vi "timestampAndDataToTable 4ch.vi"(7 "show time left [F]":bool, 9 "device type [AB1004]":T2=1004 items=["any"=0, "AB1002"=1002, "AB1004"=1004], 10 "data in":T4(array[cluster]), 11 "session start timestamp":timestamp) -> (1 "table data":string[][](array[string]), 2 "table headers":string[](array[string]), 3 "read timestamp":timestamp[](array[timestamp]))   [LabVIEW 2015]
doc: "Arranges data from queue in a 2D string array to be written or displayed as a table.\nData from queue is an array with counter4ch data clusters and their timestamps.\nRemoves the time_left column if requested."
uses:
  <instrlib>/Tausand AB1000/Public/Controls/counters4ch.ctl
  <instrlib>/Tausand AB1000/Public/Controls/deviceTypeRing.ctl
  <instrlib>/Tausand AB1000/Public/Controls/counters2ch.ctl
  <instrlib>/Tausand AB1000/Tausand AB1000.lvlib
panel:
  out "col index to remove":i32[](array[numeric])
  out "erase this col":bool
  in  "counters":T1
  out "time from begin in s":string[](array[string])
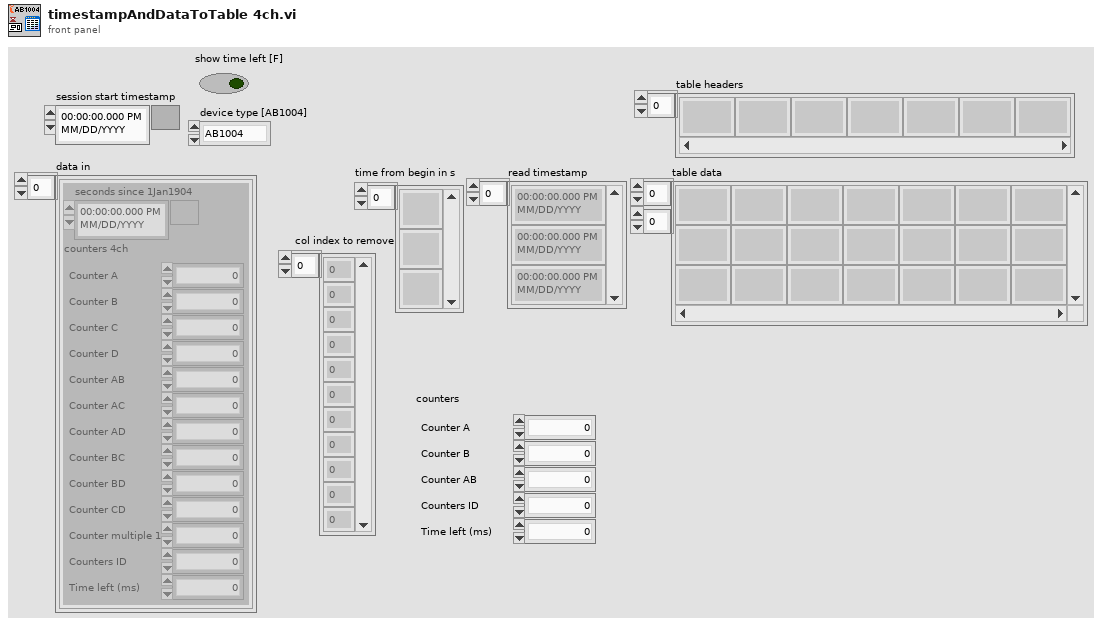
[diagram p1: front panel]
types:
  T1 = typedef "Tausand AB1000.lvlib/counters2ch.ctl" = cluster{"counter_A":u32, "counter_B":u32, "counter_AB":u32, "counters_ID":u32, "time_left":u32}
  T2 = typedef "Tausand AB1000.lvlib/deviceTypeRing.ctl" = u16
  T3 = typedef "Tausand AB1000.lvlib/counters4ch.ctl" = cluster{"counter_A":u32, "counter_B":u32, "counter_C":u32, "counter_D":u32, "counter_AB":u32, "counter_AC":u32, "counter_AD":u32, "counter_BC":u32, "counter_BD":u32, "counter_CD":u32, "counter_multiple_1":u32, "counters_ID":u32, "time_left":u32}
  T4 = cluster{"seconds since 1Jan1904":timestamp, "counters 4ch":T3}[]
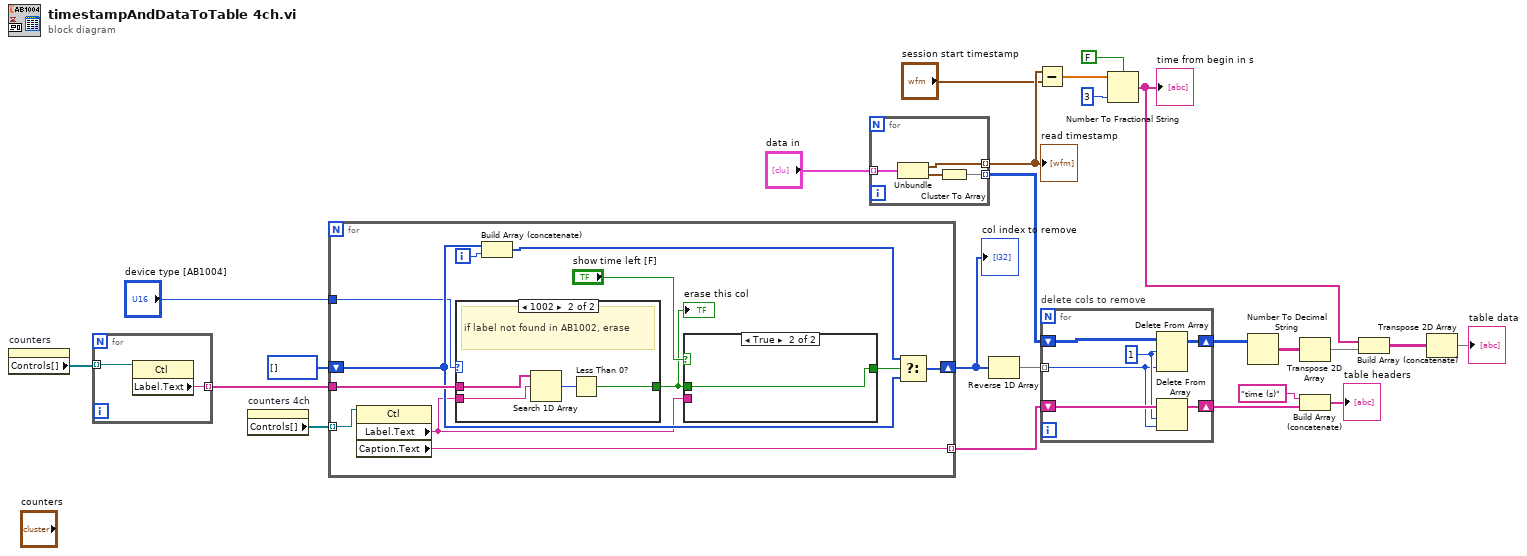
[diagram p0: block diagram]
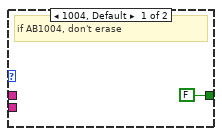
[diagram p2: hidden frame]
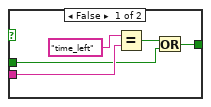
[diagram p3: hidden frame]
diagram:
  n1 = property on="counters" class="Clust (strict)"() -> ("Controls[]"=w1:refnum<vi>[])  [unwired: 2 in, 2 out]
  n2 = for {
    tunnel: w1 -> [w26] mode=indexing
    tunnel: [w25] -> w10 mode=indexing
    n3 = property class="Ctl"(reference=w26) -> ("Label.Text"=w25:string)  [unwired: 1 in, 2 out]
  }
  n4 = property on="counters 4ch" class="Clust (strict)"() -> ("Controls[]"=w15:refnum<vi>[])  [unwired: 2 in, 2 out]
  n5 = for {
    tunnel: w15 -> [w38] mode=indexing
    tunnel: [w27] -> w4 mode=indexing
    tunnel: w10 -> [w37]
    shift-right: [w33] -> w7
    shift-left: i32[] [] -> [w34]
    tunnel: "device type [AB1004]" -> [w29]
    i -> [w36]
    n6 = property class="Ctl"(reference=w38) -> ("Label.Text"=w28:string, "Caption.Text"=w27:string)  [unwired: 1 in, 2 out]
    n7 = case shown="1002" w29 {
      tunnel: w37 -> [_ w43]
      tunnel: w28 -> [_ w41]
      tunnel: [FALSE w40] -> w31
      frame 1004, Default {
        # "if AB1004, don't erase"
      }
      frame 1002 {
        # "if label not found in AB1002, erase"
        n8 = Search 1D Array(1D array=w43, element=w41) -> (index of element=w42:i32)  [unwired: 1 in]
        n9 = Less Than 0?(x=w42) -> (x < 0?=w40:bool)
      }
    }
    "erase this col" <- w31
    n10 = Build Array (concatenate)(w34, w36) -> (w35:i32[])
    n11 = case shown="True" "show time left [F]" {
      tunnel: w28 -> [w48 _]
      tunnel: [w44 w49] -> w30
      tunnel: w31 -> [w45 w49]
      frame False {
        n12 = Equal?(x="time_left" ("element"), y=w48) -> (x = y?=w46:bool)
        n13 = Or(x=w46, y=w45) -> (x .or. y?=w44:bool)
      }
      frame True {
      }
    }
    n14 = Select(t=w35, s=w30, f=w34) -> (s? t:f=w33:i32[])
  }
  "col index to remove" <- w7
  n15 = for {
    tunnel: "data in" -> [w53] mode=indexing
    tunnel: [w52] -> w22 mode=indexing
    tunnel: [w51] -> w8 mode=indexing
    n16 = Unbundle(w53) -> ("seconds since 1Jan1904"=w52:timestamp, "counters 4ch"=w50:T3)
    n17 = Cluster To Array(cluster=w50) -> (array=w51:u32[])
  }
  "read timestamp" <- w22
  n18 = Reverse 1D Array(array=w7) -> (reversed array=w5:i32[])
  n19 = Subtract(x=w22, y="session start timestamp") -> (x-y=w19:dbl[])
  n20 = for "delete cols to remove" {
    tunnel: w5 -> [w54] mode=indexing
    shift-right: [w58] -> w2
    shift-left: w8 -> [w59]
    shift-right: [w56] -> w3
    shift-left: w4 -> [w57]
    w55 = 1 ("length")
    n21 = Delete From Array(array=w59, length=w55, index (col)=w54) -> (array with subset deleted=w58:u32[][])  [unwired: 1 in, 1 out]
    n22 = Delete From Array(array=w57, length=w55, index=w54) -> (array with subset deleted=w56:string[])  [unwired: 1 out]
  }
  n23 = Number To Fractional String(use system decimal point (T)=FALSE, number=w19, precision (6)=i16 3) -> (F-format string=w18:string[])  [unwired: 1 in]
  "time from begin in s" <- w18
  n24 = Number To Decimal String(number=w2) -> (decimal integer string=w14:string[][])  [unwired: 1 in]
  n25 = Transpose 2D Array(2D array=w14) -> (transposed array=w13:string[][])
  n26 = Build Array (concatenate)("time (s)" ("Caption.Text"), w3) -> (→"table headers":string[])
  n27 = Build Array (concatenate)(w18, w13) -> (w24:string[][])
  n28 = Transpose 2D Array(2D array=w24) -> (transposed array=→"table data":string[][])
